vi "TextSearchTips.vi"() -> ()   [LabVIEW 2023]
panel:
  out "Result array":string[](array[string])
  in  "stop":bool
  out "size(s)":i32
  out "Results":string[](array[string])
  in  "This Word":string
  in  "Text":string
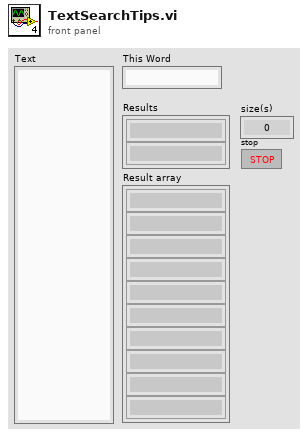
[diagram p1: front panel]
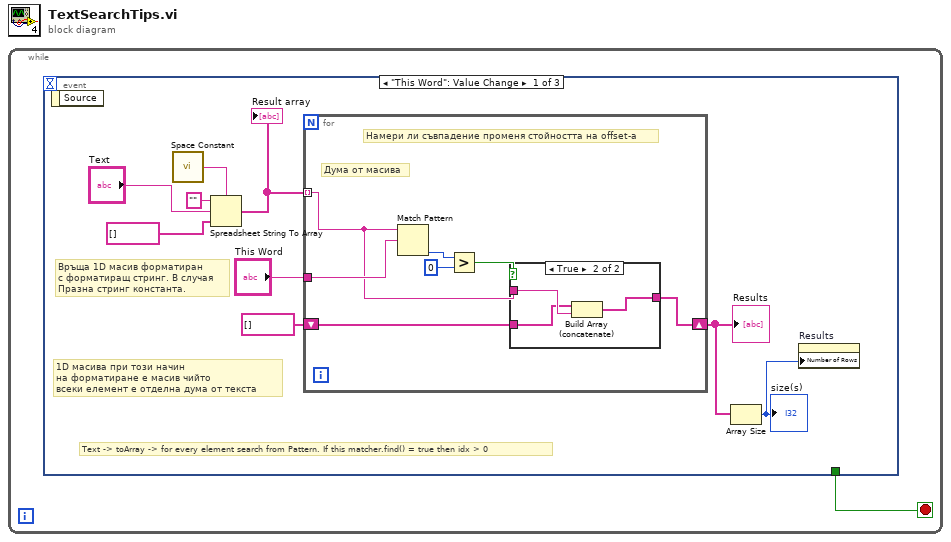
[diagram p0: block diagram]
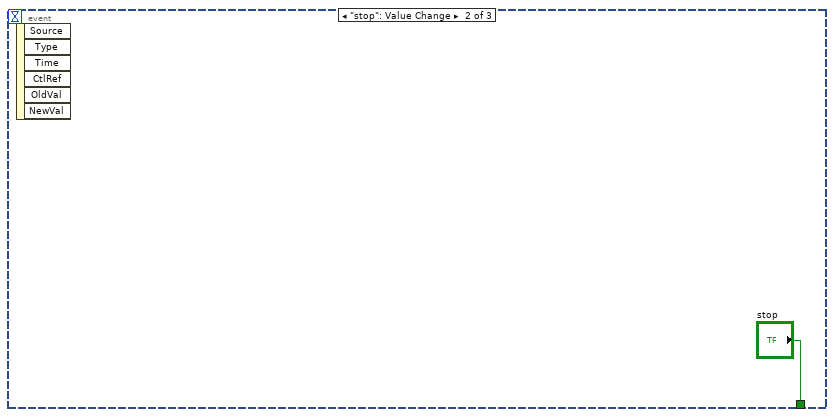
[diagram p3: hidden frame]
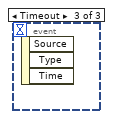
[diagram p4: hidden frame]
diagram:
  n1 = while {
    stop <- w1 stop-if-true
    n2 = event shown="[0] \"This Word\": Value Change" {
      selector: _ -> [_ _ _]
      dyn-events: _ -> [_ _ _]
      timeout: _ -> [_ _ _]
      tunnel: [_ "stop" _] -> w1
      event "This Word": Value Change {
        # "Text -> toArray -> for every element search from Pattern. If this matcher.find() = true then idx > 0"
        # "1D масива при този начин\nна форматиране е масив чийто\nвсеки елемент е отделна дума от текста"
        # "Връща 1D масив форматиран\nс форматиращ стринг. В случая\nПразна стринг константа."
        n3 = event-data() -> ()  [unwired: 1 in, 1 out]
        n4 = call <vilib>:"Space Constant.vi"() -> ("String"=w9:string)
        n5 = Spreadsheet String To Array(delimiter (Tab)=w9, format string="", spreadsheet string="Text", array type (2D Dbl)=string[] []) -> (array=w2:string[])
        "Result array" <- w2
        n6 = for {
          tunnel: w2 -> [w11] mode=indexing
          tunnel: "This Word" -> [w14]
          shift-right: [w13] -> w4
          shift-left: string[] [] -> [w12]
          # "Дума от масива"
          # "Намери ли съвпадение променя стойността на offset-a"
          n7 = Match Pattern(string=w11, regular expression=w14) -> (offset past match=w17:i32)  [unwired: 1 in, 3 out]
          n8 = Greater?(x=w17, y=0) -> (0:w15:bool)
          n9 = case shown="True" w15 {
            tunnel: w11 -> [_ w21]
            tunnel: [w18 w20] -> w13
            tunnel: w12 -> [w18 w19]
            frame False {
            }
            frame True {
              n10 = Build Array (concatenate)(w19, w21) -> (w20:string[])
            }
          }
        }
        "Results" <- w4
        n11 = Array Size(array=w4) -> (size(s)=w3:i32)
        "size(s)" <- w3
        n12 = property on="Results" class="Arr (strict)"("Number of Rows"=w3) -> ()  [unwired: 2 in, 2 out]
      }
      event "stop": Value Change {
        n13 = event-data() -> ()  [unwired: 1 in, 6 out]
      }
      event Timeout {
        n14 = event-data() -> ()  [unwired: 1 in, 3 out]
      }
    }
  }
